vi "Enable PWM.vi"(7 "node-ID":u8, 8 "error in (no error)":errorcluster, 11 "interface object in":refnum<k20>) -> (0 "error out":errorcluster, 3 "interface object out":refnum<k20>)   [LabVIEW 2016]
uses:
  <vilib>/CANopenLib/CANOPEN.llb/CANopen RPDO Create.vi
  <vilib>/CANopenLib/CANOPEN.llb/CANopen RPDO Close.vi
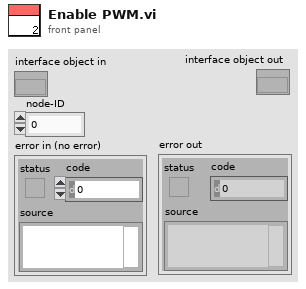
[diagram p1: front panel]
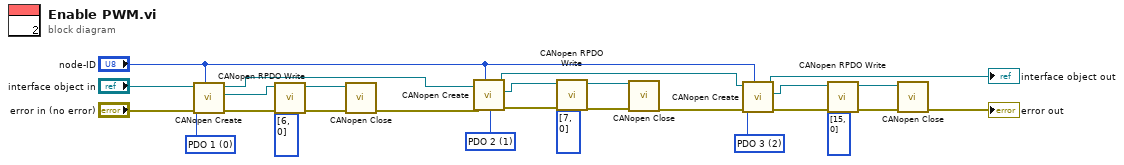
[diagram p0: block diagram]
diagram:
  w18 = u8 2 items=["PDO 1", "PDO 2", "PDO 3", "PDO 4"] ("PDO channel")
  w19 = u8 1 items=["PDO 1", "PDO 2", "PDO 3", "PDO 4"] ("PDO channel")
  w24 = u8 0 items=["PDO 1", "PDO 2", "PDO 3", "PDO 4"] ("PDO channel")
  n1 = call-poly <vilib>:"CANopen Create.vi"("node-ID"="node-ID", "error in (no error)"="error in (no error)", "PDO channel"=w24, "interface object in"="interface object in") -> ("error out"=w26:errorcluster, "RPDO object out"=w27:refnum<k20>, "interface object out"=w6:refnum<k20>)  [unwired: 5 in]
  n2 = call <vilib>:"CANopen RPDO Write.vi"("error in (no error)"=w26, "data"=u8[] [6, 0], "RPDO object in"=w27) -> ("error out"=w12:errorcluster, "RPDO object out"=w13:refnum<k20>)  [unwired: 7 in]
  n3 = call-poly <vilib>:"CANopen Close.vi"("error in (no error)"=w12, "RPDO object in"=w13) -> ("error out"=w7:errorcluster)  [unwired: 9 in]
  n4 = call-poly <vilib>:"CANopen Create.vi"("node-ID"="node-ID", "error in (no error)"=w7, "PDO channel"=w19, "interface object in"=w6) -> ("error out"=w17:errorcluster, "RPDO object out"=w16:refnum<k20>, "interface object out"=w4:refnum<k20>)  [unwired: 5 in]
  n5 = call <vilib>:"CANopen RPDO Write.vi"("error in (no error)"=w17, "data"=u8[] [7, 0], "RPDO object in"=w16) -> ("error out"=w10:errorcluster, "RPDO object out"=w11:refnum<k20>)  [unwired: 7 in]
  n6 = call-poly <vilib>:"CANopen Close.vi"("error in (no error)"=w10, "RPDO object in"=w11) -> ("error out"=w5:errorcluster)  [unwired: 9 in]
  n7 = call-poly <vilib>:"CANopen Create.vi"("node-ID"="node-ID", "error in (no error)"=w5, "PDO channel"=w18, "interface object in"=w4) -> ("error out"=w14:errorcluster, "RPDO object out"=w15:refnum<k20>, "interface object out"=→"interface object out":refnum<k20>)  [unwired: 5 in]
  n8 = call <vilib>:"CANopen RPDO Write.vi"("error in (no error)"=w14, "data"=u8[] [15, 0], "RPDO object in"=w15) -> ("error out"=w8:errorcluster, "RPDO object out"=w9:refnum<k20>)  [unwired: 7 in]
  n9 = call-poly <vilib>:"CANopen Close.vi"("error in (no error)"=w8, "RPDO object in"=w9) -> ("error out"=→"error out":errorcluster)  [unwired: 9 in]
